vi "Check Channel Pairs (SubVI).vi"(5 "seconds to wait":u32=100, 7 "Test Values":dbl[](array[numeric]), 8 "error in (no error)":errorcluster, 9 "Scalar Input Aliases":string[](array[string]), 10 "Scalar Output Aliases":string[](array[string]), 11 ".NET Refnum in":T1) -> (0 "error out":errorcluster, 1 "Input Scalar Channel Values":dbl[](array[numeric]), 2 "Output Scalar Channel Values":dbl[](array[numeric]), 3 ".NET Refnum out":T1)   [LabVIEW 2023, in "FPGA Addon Test Class.lvclass"]
uses:
  FPGA Addon Test Class.lvclass
  <vilib>/NI VeriStand/Execution/Workspace/WorkspaceAPI.ctl
  <vilib>/NI VeriStand/Execution/Workspace/NI_VS Workspace ExecutionAPI.lvlib
  NationalInstruments.VeriStand.ClientAPI
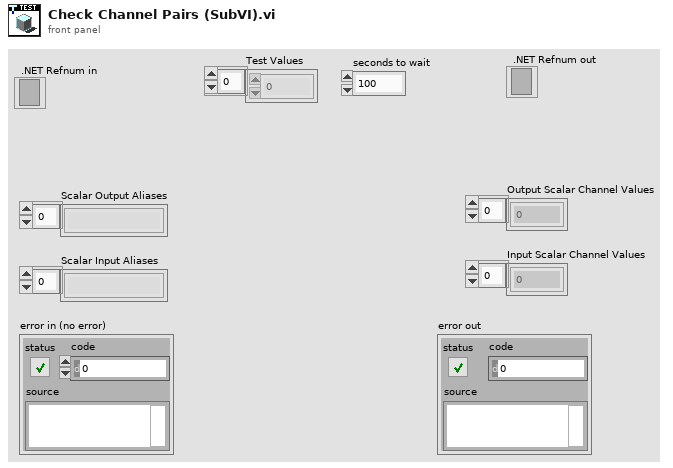
[diagram p1: front panel]
types:
  T1 = typedef "NI_VS Workspace ExecutionAPI.lvlib/WorkspaceAPI.ctl" = refnum<k24>
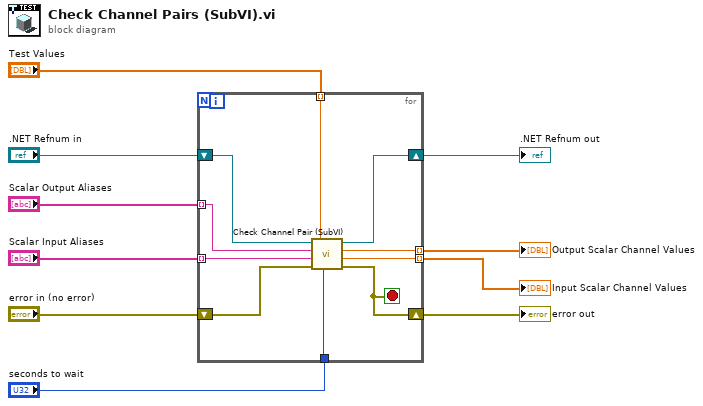
[diagram p0: block diagram]
diagram:
  n1 = for {
    tunnel: "Scalar Output Aliases" -> [w19] mode=indexing
    tunnel: "Scalar Input Aliases" -> [w18] mode=indexing
    tunnel: "Test Values" -> [w20] mode=indexing
    tunnel: [w17] -> w7 mode=indexing
    tunnel: [w16] -> w6 mode=indexing
    shift-right: [w14] -> w9
    shift-left: "error in (no error)" -> [w15]
    tunnel: "seconds to wait" -> [w11]
    shift-right: [w12] -> w1
    shift-left: ".NET Refnum in" -> [w13]
    stop <- w14 stop-if-true
    n2 = call "Check Channel Pair (SubVI).vi"("seconds to wait"=w11, "OutputChannel Value in"=w20, "error in (no error)"=w15, "Input Channel"=w18, "Output Channel"=w19, "WorkspaceManager in"=w13) -> ("error out"=w14:errorcluster, "OutputChannel Value out"=w16:dbl, "InputChanel Value"=w17:dbl, "WorkspaceManager out"=w12:T1)  [unwired: 2 in]
  }
  "error out" <- w9
  "Output Scalar Channel Values" <- w7
  "Input Scalar Channel Values" <- w6
  ".NET Refnum out" <- w1
